vi "Read Error Queue.vi"(8 "error in (no error)":errorcluster, 11 "VISA resource name":refnum<visa-resource-name>) -> (0 "error out":errorcluster, 1 "errors read":u8, 2 "error queue":string, 3 "VISA resource name out":refnum<visa-resource-name>)   [LabVIEW 2018, in "Agilent 87XX Series.lvlib"]
doc: "This VI is used to read and clear the HP8753B's error queue. The error queue can hold up to 20 errors. Each error message can be up to 50 characters. If there are no errors in the queue or all the the errors have been read out, the message ' 0,\"NO ERRORS\" ' will be displayed."
uses:
  Agilent 87XX Series.lvlib
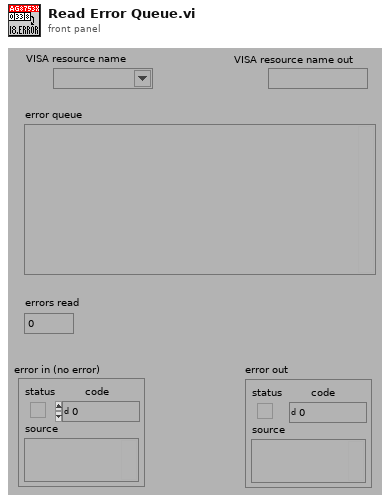
[diagram p1: front panel]
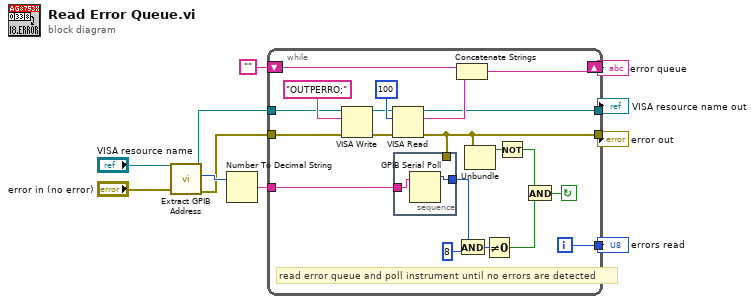
[diagram p0: block diagram]
diagram:
  n1 = call "Extract GPIB Address.VI"("error in (no error)"="error in (no error)", "VISA resource name"="VISA resource name") -> ("error out"=w4:errorcluster, "GPIB address"=w5:u16, "VISA resource name out"=w2:refnum<visa-resource-name>)  [unwired: 6 in, 1 out]
  n2 = Number To Decimal String(number=w5) -> (decimal integer string=w6:string)  [unwired: 1 in]
  n3 = while {
    tunnel: w6 -> [w19]
    tunnel: w4 -> [w21]
    tunnel: w2 -> [w22]
    tunnel: [w18] -> w7
    tunnel: [w23] -> w8
    tunnel: [w27] -> w9
    shift-left: "" -> [w31]
    shift-right: [w30] -> w10
    i -> [w27]
    stop <- w14 continue-if-true
    # "read error queue and poll instrument until no errors are detected"
    n4 = VISA Write(VISA resource name=w22, write buffer="OUTPERRO;", error in (no error)=w21) -> (VISA resource name out=w12:refnum<visa-resource-name>, error out=w26:errorcluster)  [unwired: 1 out]
    n5 = VISA Read(VISA resource name=w12, byte count=u32 100, error in (no error)=w26) -> (VISA resource name out=w23:refnum<visa-resource-name>, read buffer=w24:string, error out=w18:errorcluster)  [unwired: 1 out]
    n6 = stacked-sequence {
      tunnel: [w33] -> w20
      tunnel: w18 -> [_]
      tunnel: w19 -> [w32]
      frame #0 {
        n7 = GPIB Serial Poll(0:w32) -> (2:w33:i16)  [unwired: 1 in, 2 out]
      }
    }
    n8 = Concatenate Strings(w31, w24) -> (w30:string)
    n9 = And(x=w20, y=i16 8) -> (x .and. y?=w28:i16)
    n10 = Unbundle(w18) -> ("status"=w17:bool)  [unwired: 2 out]
    n11 = Not Equal To 0?(x=w28) -> (x != 0?=w15:bool)
    n12 = Not(x=w17) -> (.not. x?=w16:bool)
    n13 = And(x=w16, y=w15) -> (x .and. y?=w14:bool)
  }
  "error queue" <- w10
  "errors read" <- w9
  "VISA resource name out" <- w8
  "error out" <- w7
